vi "clear PF.vi"(10 "引用":refnum<vi>) -> (2 "引用输出":refnum<vi>)   [LabVIEW 2018]
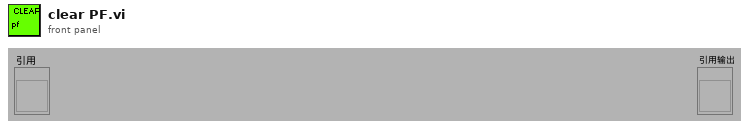
[diagram p1: front panel]
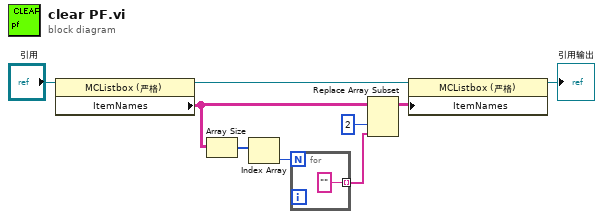
[diagram p0: block diagram]
diagram:
  n1 = property class="MCListbox (严格)"(reference="引用") -> (reference out=w4:refnum<vi>, "ItemNames"=w7:string[][])  [unwired: 1 in, 1 out]
  n2 = Array Size(array=w7) -> (size(s)=w9:i32[])
  n3 = Index Array(array=w9) -> (element=w8:i32)  [unwired: 1 in]
  n4 = for {
    N: w8 -> [_]
    tunnel: [""] -> w5 mode=indexing
  }
  n5 = Replace Array Subset(array=w7, new element=w5, index (col)=2 ("禁用的索引 (列)")) -> (w3:string[][])  [unwired: 1 in]
  n6 = property class="MCListbox (严格)"(reference=w4, "ItemNames"=w3) -> (reference out=→"引用输出":refnum<vi>)  [unwired: 1 in, 1 out]
